vi "ProcAndStates.vi"(0 "spreadsheet string":string) -> (1 "PROCESSES":string[](array[string]), 2 "STATES":string[][](array[string]))   [LabVIEW 2009]
panel:
  out "size(s)":i32[](array[numeric])
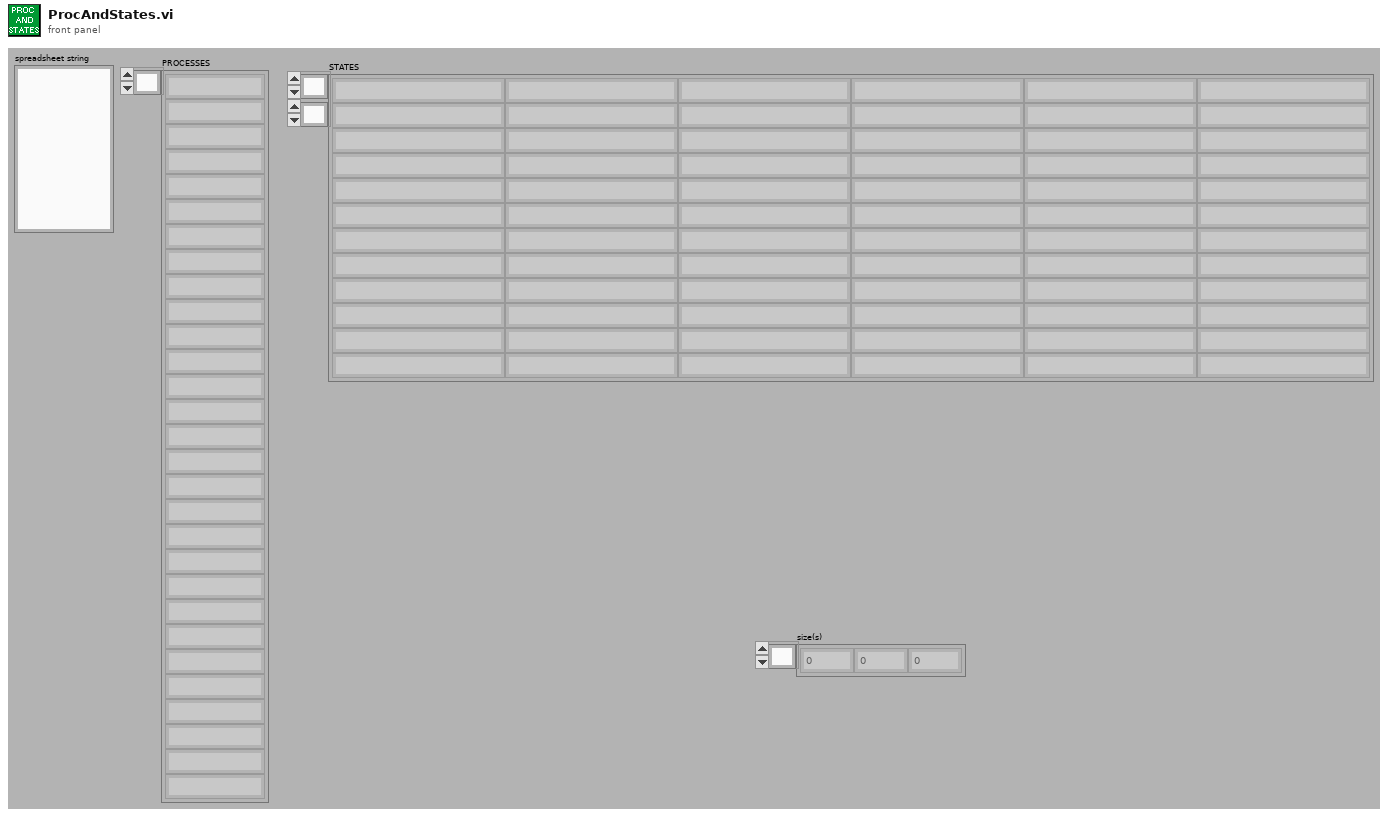
[diagram p1: front panel]
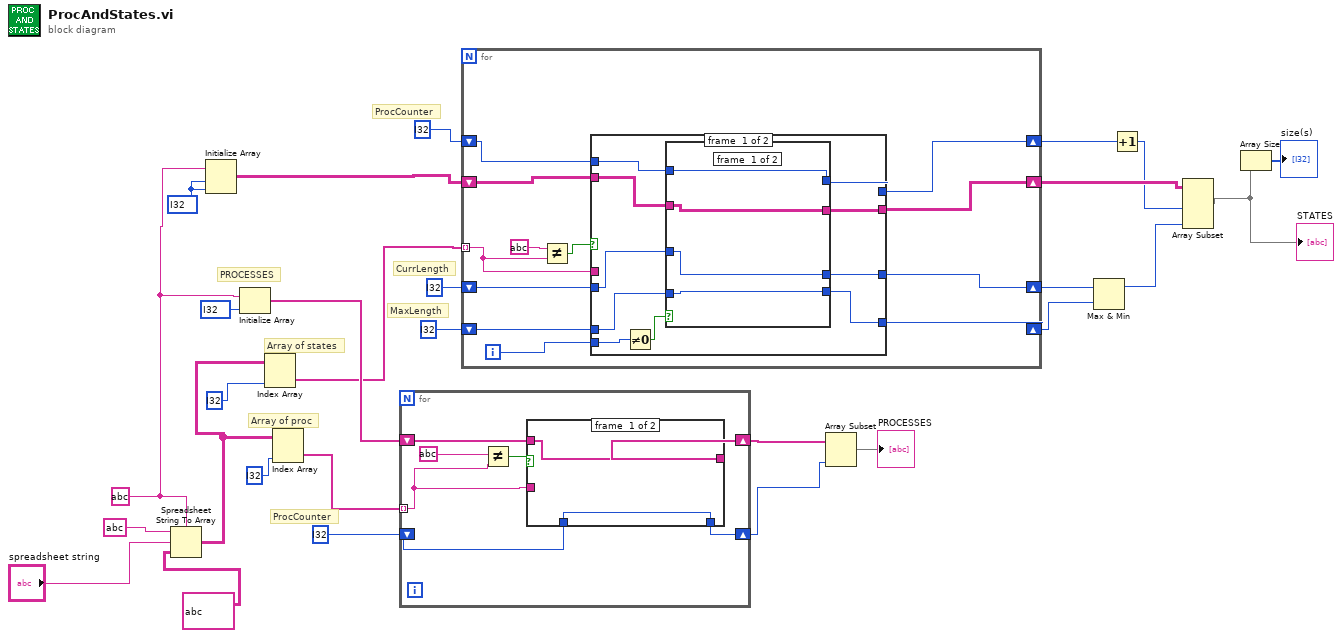
[diagram p0: block diagram]
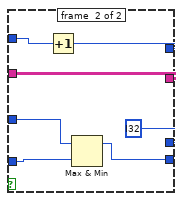
[diagram p2: hidden frame]
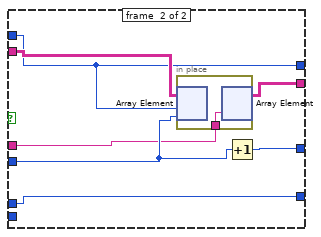
[diagram p3: hidden frame]
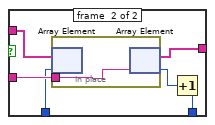
[diagram p4: hidden frame]
diagram:
  w15 = i32 ? ("dimension size")
  w16 = string ? ("delimiter (Tab)")
  # "ProcCounter"
  # "PROCESSES"
  # "CurrLength"
  # "MaxLength"
  # "ProcCounter"
  # "Array of proc"
  # "Array of states"
  n1 = Spreadsheet String To Array(delimiter (Tab)=w16, format string=string ?, spreadsheet string="spreadsheet string", array type (2D Dbl)=string[][] ?) -> (array=w27:string[][])
  n2 = Initialize Array(w16, w15, w15) -> (w20:string[][])
  n3 = Initialize Array(w16, i32 ? ("dimension size")) -> (w23:string[])
  n4 = Index Array(array=w27, index (col)=i32 ? ("index (row)")) -> (element=w17:string[])  [unwired: 1 in]
  n5 = Index Array(array=w27, index (col)=i32 ? ("index (row)")) -> (element=w22:string[])  [unwired: 1 in]
  n6 = for {
    tunnel: w22 -> [w34] mode=indexing
    shift-right: [w32] -> w9
    shift-left: w23 -> [w33]
    shift-right: [w29] -> w6
    shift-left: i32 ? ("dimension size") -> [w30]
    n7 = Not Equal?(x=string ?, y=w34) -> (x != y?=w35:bool)
    n8 = case shown="True" w35 {
      tunnel: w34 -> [_ w42]
      tunnel: w33 -> [w37 w43]
      tunnel: [w37 w38] -> w32
      tunnel: w30 -> [w36 w41]
      tunnel: [w36 w39] -> w29
      frame #0 {
      }
      frame #1 {
        n9 = in-place {
          in-place-border: w42 -> [w44]
          n10 = in-place-array #1(w43, w41) -> ()  [unwired: 1 out]
          n11 = in-place-array #1(w44) -> (w38:string[], w40:i32)
        }
        n12 = Increment(x=w40) -> (x+1=w39:i32)
      }
    }
  }
  n13 = for {
    tunnel: w17 -> [w54] mode=indexing
    shift-right: [w50] -> w2
    shift-left: w20 -> [w55]
    shift-right: [w52] -> w13
    shift-left: i32 ? ("dimension size") -> [w53]
    shift-right: [w49] -> w11
    shift-left: i32 ? ("dimension size") -> [w51]
    shift-right: [w45] -> w12
    shift-left: i32 ? ("dimension size") -> [w46]
    i -> [w47]
    n14 = Not Equal?(x=string ?, y=w54) -> (x != y?=w56:bool)
    n15 = case shown="True" w56 {
      tunnel: [w65 w81] -> w50
      tunnel: w55 -> [w66 w82]
      tunnel: w54 -> [_ w79]
      tunnel: w53 -> [w64 w78]
      tunnel: [w57 w78] -> w52
      tunnel: w51 -> [w63 w84]
      tunnel: [w62 w84] -> w49
      tunnel: w47 -> [w61 _]
      tunnel: w46 -> [w59 w80]
      tunnel: [w58 w83] -> w45
      frame #0 {
        n16 = Not Equal To 0?(x=w61) -> (x != 0?=w60:bool)
        n17 = case shown="True" w60 {
          tunnel: w66 -> [w70 w73]
          tunnel: [w70 w73] -> w65
          tunnel: w64 -> [w68 w77]
          tunnel: [w68 w72] -> w57
          tunnel: w63 -> [w69 w76]
          tunnel: [w69 w71] -> w62
          tunnel: w59 -> [w67 w75]
          tunnel: [w67 i32 ?] -> w58
          frame #0 {
          }
          frame #1 {
            n18 = Increment(x=w77) -> (x+1=w72:i32)
            n19 = Max & Min(x=w75, y=w76) -> (max(x,y)=w71:i32)  [unwired: 1 out]
          }
        }
      }
      frame #1 {
        n20 = in-place {
          in-place-border: w79 -> [w85]
          n21 = in-place-array #2(w82, w78, w80) -> ()  [unwired: 1 out]
          n22 = in-place-array #2(w85) -> (w81:string[][])  [unwired: 2 out]
        }
        n23 = Increment(x=w80) -> (x+1=w83:i32)
      }
    }
  }
  n24 = Array Subset(array=w9, length=w6) -> (→"PROCESSES":string[])  [unwired: 1 in]
  n25 = Max & Min(x=w12, y=w11) -> (max(x,y)=w5:i32)  [unwired: 1 out]
  n26 = Increment(x=w13) -> (x+1=w1:i32)
  n27 = Array Subset(array=w2, length (row)=w1, length (col)=w5) -> (w4:string[][])  [unwired: 2 in]
  "STATES" <- w4
  n28 = Array Size(array=w4) -> (size(s)=→"size(s)":i32[])
